vi "Calculate Tick Value.vi"(9 "Logarithm?":bool, 10 "Tick Count":u16, 11 "Axis Range":cluster{"Max":sgl, "Min":sgl}) -> (1 "Logarithm?":bool, 2 "Tick Value Array":sgl[](array[numeric]))   [LabVIEW 2020, in "3D Plot.lvclass"]
uses:
  3D Plot.lvclass
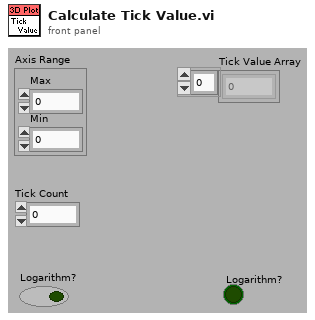
[diagram p1: front panel]
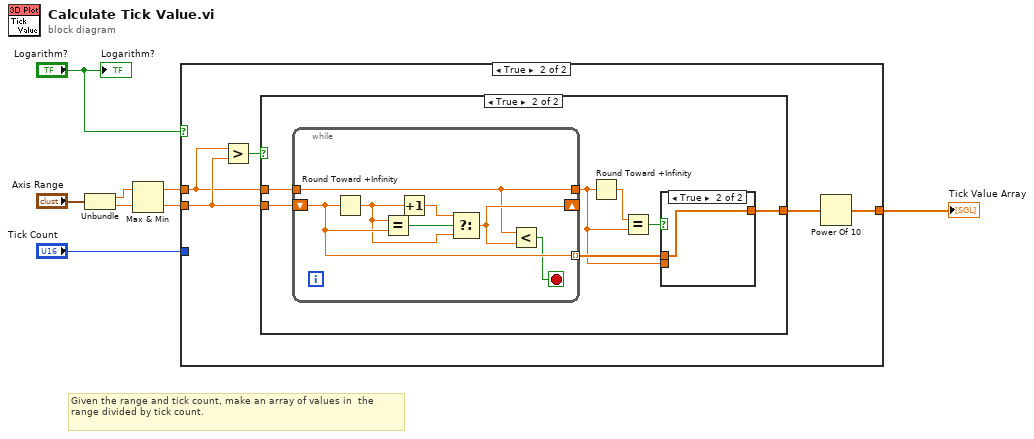
[diagram p0: block diagram]
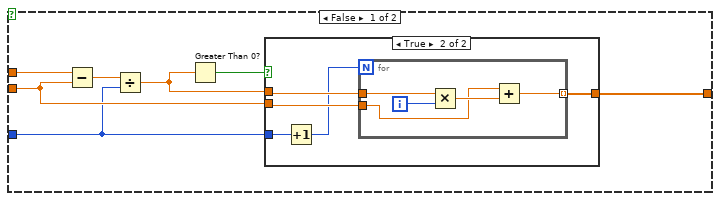
[diagram p2: hidden frame]
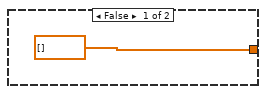
[diagram p3: hidden frame]
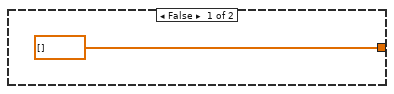
[diagram p4: hidden frame]
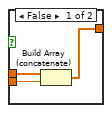
[diagram p5: hidden frame]
diagram:
  # "Given the range and tick count, make an array of values in  the range divided by tick count."
  n1 = Unbundle("Axis Range") -> ("Max"=w5:sgl, "Min"=w6:sgl)
  n2 = Max & Min(x=w5, y=w6) -> (max(x,y)=w7:sgl, min(x,y)=w8:sgl)
  n3 = case shown="True" "Logarithm?" {
    tunnel: w8 -> [w13 w29]
    tunnel: w7 -> [w12 w27]
    tunnel: [w11 w30] -> w3
    tunnel: "Tick Count" -> [w10 _]
    frame False {
      n4 = Subtract(x=w12, y=w13) -> (x-y=w14:sgl)
      n5 = Divide(x=w14, y=w10) -> (x/y=w15:sgl)
      n6 = Greater Than 0?(x=w15) -> (x > 0?=w9:bool)
      n7 = case shown="True" w9 {
        tunnel: w15 -> [_ w21]
        tunnel: w13 -> [_ w20]
        tunnel: [sgl[] [] w19] -> w11
        tunnel: w10 -> [_ w17]
        frame False {
        }
        frame True {
          n8 = Increment(x=w17) -> (x+1=w18:u16)
          n9 = for {
            N: w18 -> [_]
            tunnel: w21 -> [w26]
            tunnel: w20 -> [w23]
            tunnel: [w22] -> w19 mode=indexing
            i -> [w25]
            n10 = Multiply(x=w26, y=w25) -> (x*y=w24:sgl)
            n11 = Add(x=w23, y=w24) -> (x+y=w22:sgl)
          }
        }
      }
    }
    frame True {
      n12 = Greater?(x=w27, y=w29) -> (0:w28:bool)
      n13 = case shown="True" w28 {
        tunnel: w29 -> [_ w39]
        tunnel: [sgl[] [] w36] -> w31
        tunnel: w27 -> [_ w34]
        frame False {
        }
        frame True {
          n14 = while {
            tunnel: w34 -> [w44]
            shift-right: [w46] -> _
            shift-left: w39 -> [w48]
            tunnel: [w48] -> w37 mode=indexing
            tunnel: [w44] -> w33
            stop <- w45 stop-if-true
            n15 = Round Toward +Infinity(x=w48) -> (ceil(x): smallest int >= x=w47:sgl)
            n16 = Equal?(x=w47, y=w48) -> (x = y?=w50:bool)
            n17 = Increment(x=w47) -> (x+1=w49:sgl)
            n18 = Select(t=w49, s=w50, f=w47) -> (s? t:f=w46:sgl)
            n19 = Less?(x=w44, y=w46) -> (x < y?=w45:bool)
          }
          n20 = Round Toward +Infinity(x=w33) -> (ceil(x): smallest int >= x=w38:sgl)
          n21 = Equal?(x=w38, y=w33) -> (x = y?=w35:bool)
          n22 = case shown="True" w35 {
            tunnel: w37 -> [w42 w43]
            tunnel: [w41 w43] -> w36
            tunnel: w33 -> [w40 _]
            frame False {
              n23 = Build Array (concatenate)(w42, w40) -> (w41:sgl[])
            }
            frame True {
            }
          }
        }
      }
      n24 = Power Of 10(x=w31) -> (10^x=w30:sgl[])
    }
  }
  "Tick Value Array" <- w3
  "Logarithm?" <- "Logarithm?"
